vi "Mode sync(pop-up).vi"(1 "Époq. in":dbl format="%.1g", 2 "Déc. in":string, 3 "RA in":string) -> (0 "Valeur":u32=1)   [LabVIEW 2011]
panel:
  out "Époque:":dbl format="%.2f"
  in  "Annuler":bool
  out "Déc.:":string
  out "RA :":string
  in  "Sync scope":bool
  in  "Sync cible":bool
  # "Utiliser cette coordonnée :"
  # "Pour synchroniser :"
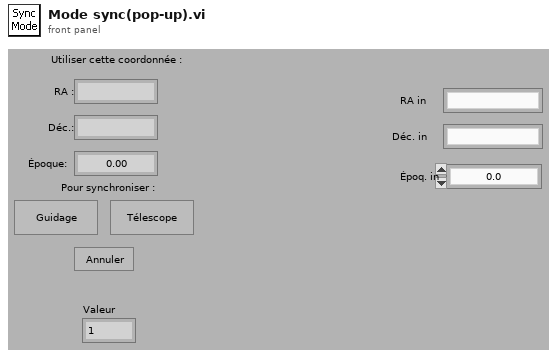
[diagram p1: front panel]
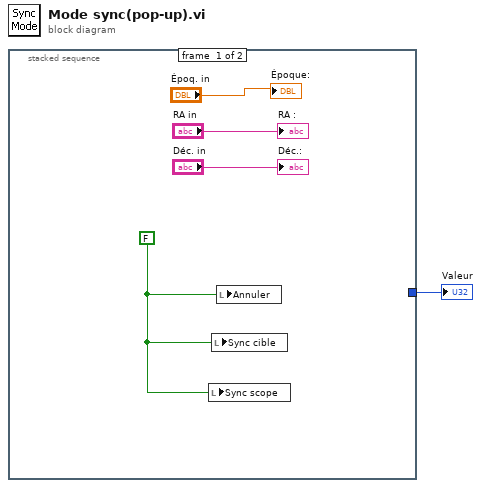
[diagram p0: block diagram]
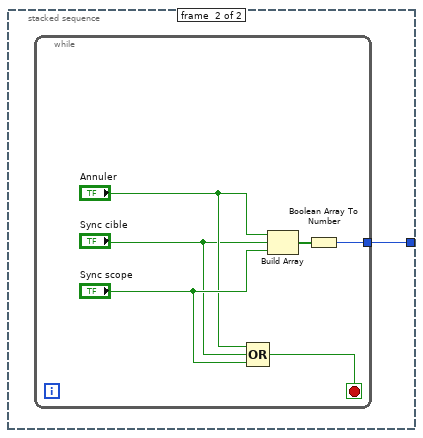
[diagram p2: hidden frame]
diagram:
  n1 = stacked-sequence {
    tunnel: [_ w6] -> w1
    frame #0 {
      w5 = FALSE
      n2 = local write "Sync scope"(w5) -> ()
      n3 = local write "Sync cible"(w5) -> ()
      n4 = local write "Annuler"(w5) -> ()
      "Déc.:" <- "Déc. in"
      "RA :" <- "RA in"
      "Époque:" <- "Époq. in"
    }
    frame #1 {
      n5 = while {
        tunnel: [w9] -> w6
        stop <- w12 stop-if-true
        n6 = Compound Arithmetic op=OR("Annuler", "Sync cible", "Sync scope") -> (w12:bool)
        n7 = Build Array("Annuler", "Sync cible", "Sync scope") -> (w10:bool[])
        n8 = Boolean Array To Number(Boolean array=w10) -> (number=w9:u32)
      }
    }
  }
  "Valeur" <- w1
